vi "LJM logger handle row modifications.vi"(4 "Row Modification Options":T2={" Row #"=1, "Delete Row"=FALSE, "Insert Row"=FALSE} {"Row #" min=1 max=2000000000}, 5 "Channel Setup":T1={"Name"=["AIN0", "AIN1", "AIN2", "AIN3", "AIN4", "AIN5", "AIN6", "AIN7", "AIN8", "AIN9", "AIN10", "AIN11", "AIN12", "AIN13", "AIN14", "AIN15", "AIN16", "AIN17", "AIN18", "AIN19", "AIN20", "AIN21", "AIN22", "AIN23", "AIN24", "AIN25", "AIN26", "AIN27", "AIN28", "AIN29", "AIN30", "AIN31", "AIN32", "AIN33", "AIN34", "AIN35", "AIN36", "AIN37", "AIN38", "AIN39", "AIN40", "AIN41", "AIN42", "AIN43", "AIN44", "AIN45", "AIN46", "AIN47", "AIN48", "AIN49", "AIN50", "AIN51", "AIN52", "AIN53", "AIN54", "AIN55", "AIN56", "AIN57", "AIN58", "AIN59", "AIN60", "AIN61", "AIN62", "AIN63", "AIN64", "AIN65", "AIN66", "AIN67", "AIN68", "AIN69", "AIN70", "AIN71", "AIN72", "AIN73", "AIN74", "AIN75", "AIN76", "AIN77", "AIN78", "AIN79", "AIN80", "AIN81", "AIN82", "AIN83", "AIN84", "AIN85", "AIN86", "AIN87", "AIN88", "AIN89", "AIN90", "AIN91", "AIN92", "AIN93", "AIN94", "AIN95", "AIN96", "AIN97", "AIN98", "AIN99"], "", "Scaling Equation"=["y=a", "y=b", "y=c", "y=d", "y=e", "y=f", "y=g", "y=h", "y=i", "y=j", "y=k", "y=l", "y=m", "y=n", "y=o", "y=p", "y=q", "y=r", "y=s", "y=t", "y=u", "y=v", "y=w", "y=x", "y=y", "y=z", "y=a2", "y=b2", "y=c2", "y=d2", "y=e2", "y=f2", "y=g2", "y=h2", "y=i2", "y=j2", "y=k2", "y=l2", "y=m2", "y=n2", "y=o2", "y=p2", "y=q2", "y=r2", "y=s2", "y=t2", "y=u2", "y=v2", "y=w2", "y=x2", "y=y2", "y=z2", "y=a3", "y=b3", "y=c3", "y=d3", "y=e3", "y=f3", "y=g3", "y=h3", "y=i3", "y=j3", "y=k3", "y=l3", "y=m3", "y=n3", "y=o3", "y=p3", "y=q3", "y=r3", "y=s3", "y=t3", "y=u3", "y=v3", "y=w3", "y=x3", "y=y3", "y=z3", "y=a4", "y=b4", "y=c4", "y=d4", "y=e4", "y=f4", "y=g4", "y=h4", "y=i4", "y=j4", "y=k4", "y=l4", "y=m4", "y=n4", "y=o4", "y=p4", "y=q4", "y=r4", "y=s4", "y=t4", "y=u4", "y=v4"], "", "Graph?"=[TRUE, TRUE, TRUE, TRUE, FALSE, FALSE, FALSE, FALSE, FALSE, FALSE, FALSE, FALSE, FALSE, FALSE, FALSE, FALSE]}) -> (2 "Channel Setup Out":T1={"Name"=["AIN0", "AIN1", "AIN2", "AIN3", "AIN4", "AIN5", "AIN6", "AIN7", "AIN8", "AIN9", "AIN10", "AIN11", "AIN12", "AIN13", "AIN14", "AIN15", "AIN16", "AIN17", "AIN18", "AIN19", "AIN20", "AIN21", "AIN22", "AIN23", "AIN24", "AIN25", "AIN26", "AIN27", "AIN28", "AIN29", "AIN30", "AIN31", "AIN32", "AIN33", "AIN34", "AIN35", "AIN36", "AIN37", "AIN38", "AIN39", "AIN40", "AIN41", "AIN42", "AIN43", "AIN44", "AIN45", "AIN46", "AIN47", "AIN48", "AIN49", "AIN50", "AIN51", "AIN52", "AIN53", "AIN54", "AIN55", "AIN56", "AIN57", "AIN58", "AIN59", "AIN60", "AIN61", "AIN62", "AIN63", "AIN64", "AIN65", "AIN66", "AIN67", "AIN68", "AIN69", "AIN70", "AIN71", "AIN72", "AIN73", "AIN74", "AIN75", "AIN76", "AIN77", "AIN78", "AIN79", "AIN80", "AIN81", "AIN82", "AIN83", "AIN84", "AIN85", "AIN86", "AIN87", "AIN88", "AIN89", "AIN90", "AIN91", "AIN92", "AIN93", "AIN94", "AIN95", "AIN96", "AIN97", "AIN98", "AIN99"], "", "Scaling Equation"=["y=a", "y=b", "y=c", "y=d", "y=e", "y=f", "y=g", "y=h", "y=i", "y=j", "y=k", "y=l", "y=m", "y=n", "y=o", "y=p", "y=q", "y=r", "y=s", "y=t", "y=u", "y=v", "y=w", "y=x", "y=y", "y=z", "y=a2", "y=b2", "y=c2", "y=d2", "y=e2", "y=f2", "y=g2", "y=h2", "y=i2", "y=j2", "y=k2", "y=l2", "y=m2", "y=n2", "y=o2", "y=p2", "y=q2", "y=r2", "y=s2", "y=t2", "y=u2", "y=v2", "y=w2", "y=x2", "y=y2", "y=z2", "y=a3", "y=b3", "y=c3", "y=d3", "y=e3", "y=f3", "y=g3", "y=h3", "y=i3", "y=j3", "y=k3", "y=l3", "y=m3", "y=n3", "y=o3", "y=p3", "y=q3", "y=r3", "y=s3", "y=t3", "y=u3", "y=v3", "y=w3", "y=x3", "y=y3", "y=z3", "y=a4", "y=b4", "y=c4", "y=d4", "y=e4", "y=f4", "y=g4", "y=h4", "y=i4", "y=j4", "y=k4", "y=l4", "y=m4", "y=n4", "y=o4", "y=p4", "y=q4", "y=r4", "y=s4", "y=t4", "y=u4", "y=v4"], "", "Graph?"=[TRUE, TRUE, TRUE, TRUE, FALSE, FALSE, FALSE, FALSE, FALSE, FALSE, FALSE, FALSE, FALSE, FALSE, FALSE, FALSE]})   [LabVIEW 2026]
uses:
  Common Logger Controls/Channel Setup.ctl
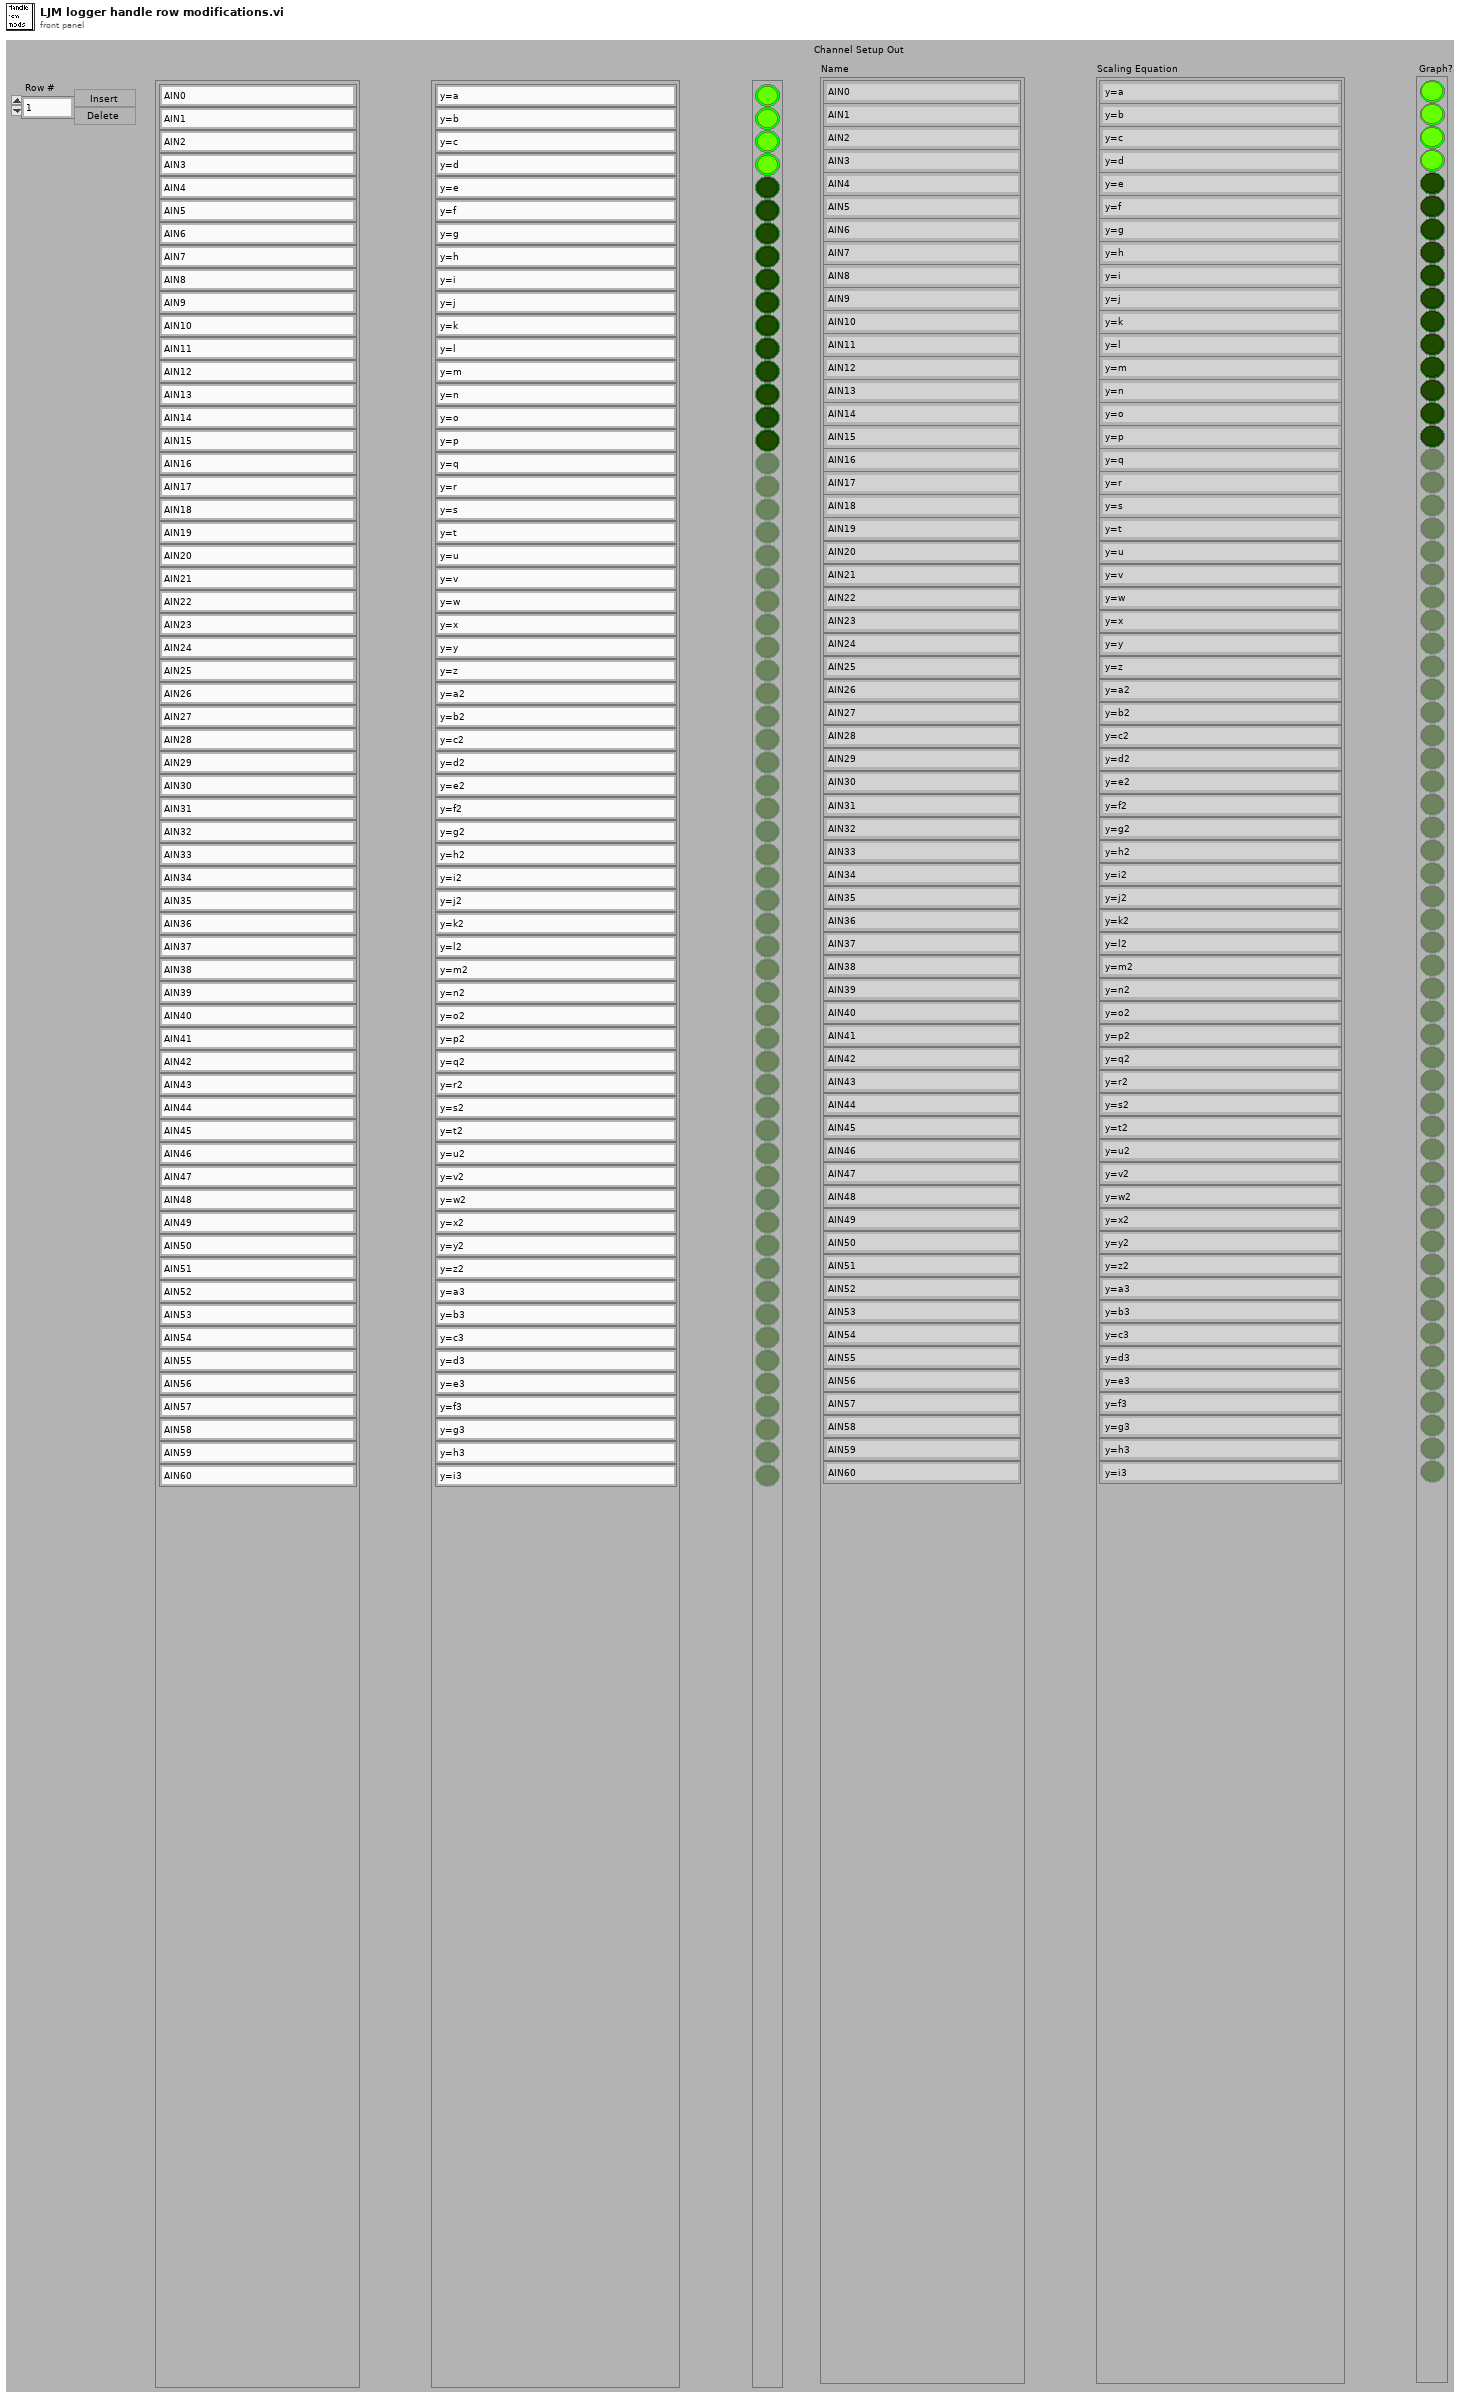
[diagram p1: front panel]
types:
  T1 = typedef "Channel Setup.ctl" = cluster{"Name":string[], string, "Scaling Equation":string[], string, "Graph?":bool[]}
  T2 = cluster{" Row #":i32, "Delete Row":bool, "Insert Row":bool}
  T3 = typedef "Program Config Cluster.ctl" = cluster{"Data File Prefix":string, "Scan Rate (Hz)":dbl, "Graph History":i32, "# Channels":i32, "Disable Scaling":bool, "Max File Size (Bytes)":i32, "Channel Setup":T1, "Interval (ms)":u32, "Write To File":bool, "Log Every n Scans":i32}
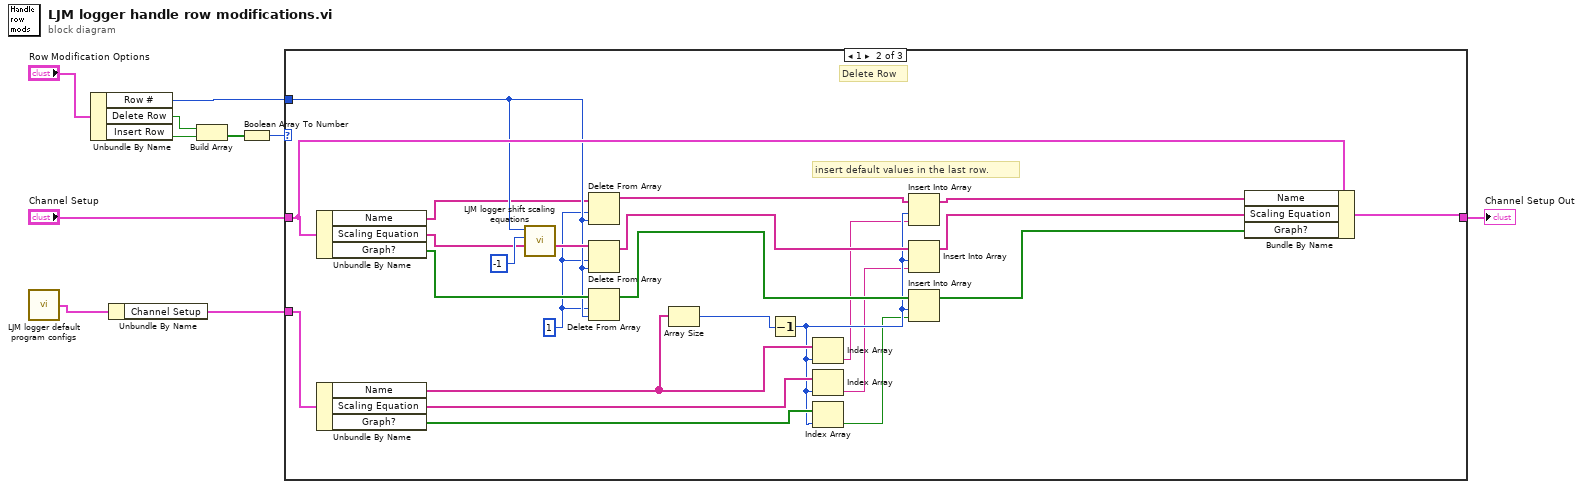
[diagram p0: block diagram]
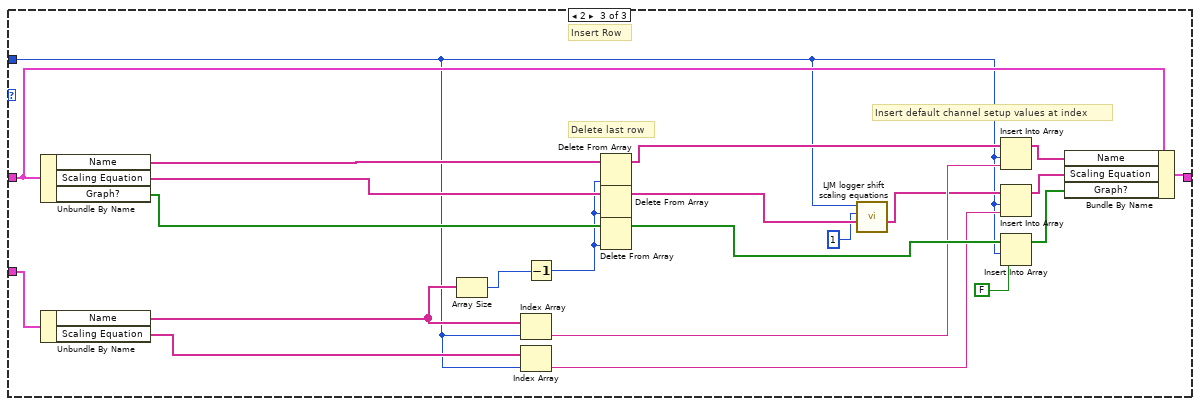
[diagram p3: hidden frame]
diagram:
  n1 = call "LJM logger default program configs.vi"() -> ("Program Configs"=w2:T3)  [unwired: 1 in]
  n2 = Unbundle By Name("Row Modification Options") -> ("Row #"=w3:i32, "Delete Row"=w8:bool, "Insert Row"=w9:bool)
  n3 = Unbundle By Name(w2) -> ("Channel Setup"=w1:T1)
  n4 = Build Array(w8, w9) -> (w7:bool[])
  n5 = Boolean Array To Number(Boolean array=w7) -> (number=w6:u32)
  n6 = case shown="1" w6 {
    tunnel: "Channel Setup" -> [w11 w30 w54]
    tunnel: [w11 w31 w53] -> w4
    tunnel: w3 -> [_ w29 w38]
    tunnel: w1 -> [_ w27 w40]
    frame 0, Default {
    }
    frame 1 {
      w28 = 1 ("length")
      # "insert default values in the last row."
      # "Delete Row"
      n7 = Unbundle By Name(w30) -> ("Name"=w16:string[], "Scaling Equation"=w34:string[], "Graph?"=w32:bool[])
      n8 = Unbundle By Name(w27) -> ("Name"=w19:string[], "Scaling Equation"=w21:string[], "Graph?"=w20:bool[])
      n9 = call "LJM logger shift scaling equations.vi"("Scaling Equations In"=w34, "Index Shift Value"=-1 ("Shift Value"), "Modification Index"=w29) -> ("Scaling Equations Out"=w33:string[])  [unwired: 3 in, 1 out]
      n10 = Delete From Array(array=w16, length=w28, index=w29) -> (array with subset deleted=w18:string[])  [unwired: 1 out]
      n11 = Delete From Array(array=w33, length=w28, index=w29) -> (array with subset deleted=w23:string[])  [unwired: 1 out]
      n12 = Delete From Array(array=w32, length=w28, index=w29) -> (array with subset deleted=w22:bool[])  [unwired: 1 out]
      n13 = Array Size(array=w19) -> (size(s)=w17:i32)
      n14 = Decrement(x=w17) -> (x-1=w15:i32)
      n15 = Index Array(array=w19, index=w15) -> (element=w14:string)
      n16 = Index Array(array=w21, index=w15) -> (element=w13:string)
      n17 = Index Array(array=w20, index=w15) -> (element=w12:bool)
      n18 = Insert Into Array(array=w18, index=w15, new element=w14) -> (w26:string[])
      n19 = Insert Into Array(array=w23, index=w15, new element=w13) -> (w25:string[])
      n20 = Insert Into Array(array=w22, index=w15, new element=w12) -> (w24:bool[])
      n21 = Bundle By Name(cluster=w30, "Name"=w26, "Scaling Equation"=w25, "Graph?"=w24) -> (w31:T1)
    }
    frame 2 {
      # "Delete last row"
      # "Insert default channel setup values at index"
      # "Insert Row"
      n22 = Unbundle By Name(w54) -> ("Name"=w52:string[], "Scaling Equation"=w57:string[], "Graph?"=w51:bool[])
      n23 = Unbundle By Name(w40) -> ("Name"=w45:string[], "Scaling Equation"=w44:string[])
      n24 = Array Size(array=w45) -> (size(s)=w37:i32)
      n25 = Index Array(array=w45, index=w38) -> (element=w48:string)
      n26 = Index Array(array=w44, index=w38) -> (element=w43:string)
      n27 = Decrement(x=w37) -> (x-1=w36:i32)
      n28 = Delete From Array(array=w52, index=w36) -> (array with subset deleted=w49:string[])  [unwired: 1 in, 1 out]
      n29 = Delete From Array(array=w57, index=w36) -> (array with subset deleted=w56:string[])  [unwired: 1 in, 1 out]
      n30 = Delete From Array(array=w51, index=w36) -> (array with subset deleted=w50:bool[])  [unwired: 1 in, 1 out]
      n31 = call "LJM logger shift scaling equations.vi"("Scaling Equations In"=w56, "Index Shift Value"=1 ("Shift Value"), "Modification Index"=w38) -> ("Scaling Equations Out"=w42:string[])  [unwired: 3 in, 1 out]
      n32 = Insert Into Array(array=w49, index=w38, new element=w48) -> (w47:string[])
      n33 = Insert Into Array(array=w42, index=w38, new element=w43) -> (w41:string[])
      n34 = Insert Into Array(array=w50, index=w38, new element=FALSE ("element")) -> (w46:bool[])
      n35 = Bundle By Name(cluster=w54, "Name"=w47, "Scaling Equation"=w41, "Graph?"=w46) -> (w53:T1)
    }
  }
  "Channel Setup Out" <- w4
